vi "dataflow.vi"() -> ()   [LabVIEW 2018]
panel:
  out "Z++":i32
  out "Z":i32
  out "Y":i32
  out "X":i32
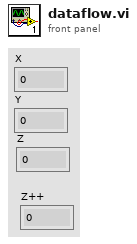
[diagram p1: front panel]
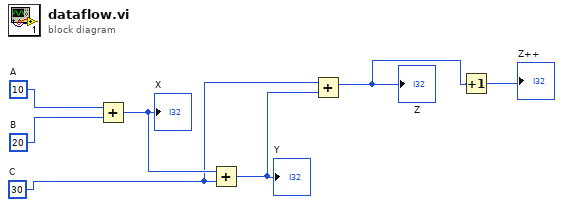
[diagram p0: block diagram]
diagram:
  w3 = 30  # C
  w6 = 20  # B
  w7 = 10  # A
  n1 = Add(x=w7, y=w6) -> (x+y=w5:i32)
  "X" <- w5
  n2 = Add(x=w5, y=w3) -> (x+y=w4:i32)
  "Y" <- w4
  n3 = Add(x=w3, y=w4) -> (x+y=w2:i32)
  "Z" <- w2
  n4 = Increment(x=w2) -> (x+1=→"Z++":i32)
